vi "test.ResumeAfterError.vi"() -> ()   [LabVIEW 2014]
uses:
  GLue.lvlib
  Private/Class/class.GLue.lvclass
panel:
  out "Numeric":i32
  in  "stop":bool
  out "Status":i32
  out "error out":errorcluster
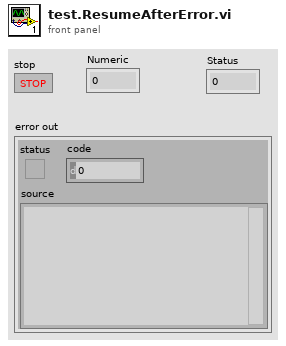
[diagram p1: front panel]
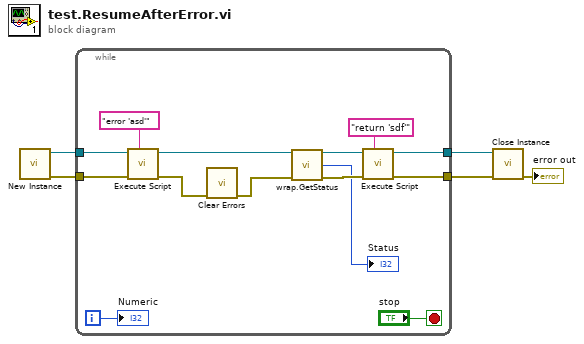
[diagram p0: block diagram]
diagram:
  n1 = call "New Instance.vi"() -> ("error out"=w5:errorcluster, "GLue out"=w4:refnum<class "class.GLue.lvclass">)  [unwired: 10 in]
  n2 = while {
    tunnel: w5 -> [w19]
    tunnel: w4 -> [w18]
    tunnel: [w16] -> w3
    tunnel: [w15] -> w2
    i -> [w6]
    stop <- "stop" stop-if-true
    n3 = call "Execute Script.vi"("Script"="error 'asd'", "error in"=w19, "GLue in"=w18) -> ("error out"=w8:errorcluster, "GLue out"=w9:refnum<class "class.GLue.lvclass">)  [unwired: 6 in, 1 out]
    n4 = call <vilib>:"Clear Errors.vi"("error in (no error)"=w8) -> ("error out"=w11:errorcluster)  [unwired: 5 in, 1 out]
    n5 = call "wrap.GetStatus.vi"("class.GLue in"=w9, "error in (no error)"=w11) -> ("class.GLue out"=w13:refnum<class "class.GLue.lvclass">, "Status"=→"Status":i32, "error out"=w12:errorcluster)  [unwired: 11 in]
    n6 = call "Execute Script.vi"("Script"="return 'sdf'", "error in"=w12, "GLue in"=w13) -> ("error out"=w15:errorcluster, "GLue out"=w16:refnum<class "class.GLue.lvclass">)  [unwired: 6 in, 1 out]
    "Numeric" <- w6
  }
  n7 = call "Close Instance.vi"("error in"=w2, "GLue in"=w3) -> ("error out"=→"error out":errorcluster)  [unwired: 9 in]
